vi "读取输入缓冲区大小.vi"(8 "error in (no error)":errorcluster caption="错误输入（无错误）", 11 "串口 输入":refnum<class "串口.lvclass"> caption="DNL_LabVIEW Object in") -> (0 "error out":errorcluster caption="错误输出", 3 "串口 输出":refnum<class "串口.lvclass"> caption="DNL_LabVIEW Object out", 10 "ReadBufferSize":i32)   [LabVIEW 2012, in "串口.lvclass"]
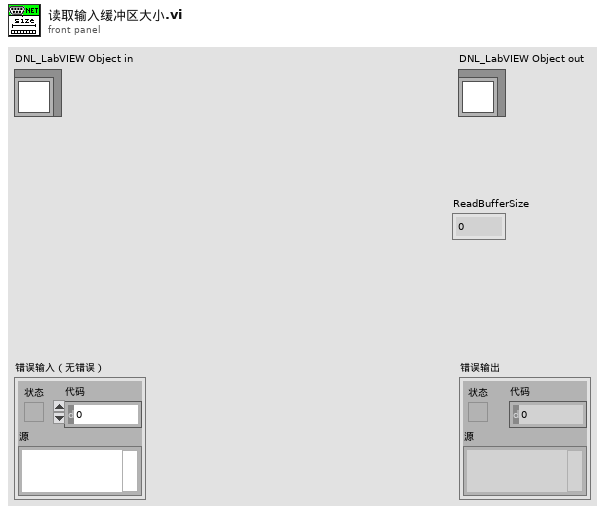
[diagram p1: front panel]
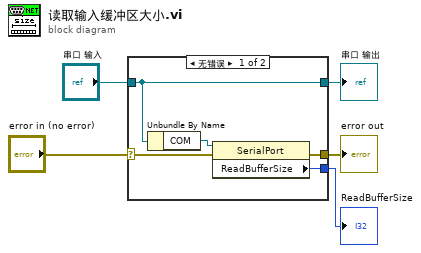
[diagram p0: block diagram]
diagram:
  n1 = case shown="无错误" "error in (no error)" {
    selector: "error in (no error)" -> [w7 w12]
    tunnel: [w6 w12] -> w4
    tunnel: [w10 w11] -> w2
    tunnel: "串口 输入" -> [w10 w11]
    tunnel: [w8 _] -> w1
    frame No Error {
      n2 = Unbundle By Name(w10) -> ("COM"=w9:refnum<k24>)
      n3 = property class="SerialPort"(reference=w9, error in=w7) -> (error out=w6:errorcluster, "ReadBufferSize"=w8:i32)  [unwired: 1 out]
    }
    frame Error {
    }
  }
  "error out" <- w4
  "串口 输出" <- w2
  "ReadBufferSize" <- w1
